vi "Delete Notebook Backup on Quit.vi"(8 "Error In":errorcluster, 11 "Main VI Name":string) -> (0 "Error Out":errorcluster)   [LabVIEW 2019, in "Notebook.lvlib"]
uses:
  Notebook.lvlib
panel:
  # "Check if the Notebook window is open:\nif it is,  don'r do anything.\nif it isn't, delete the backup.\n\nCall this VI when quitting your application."
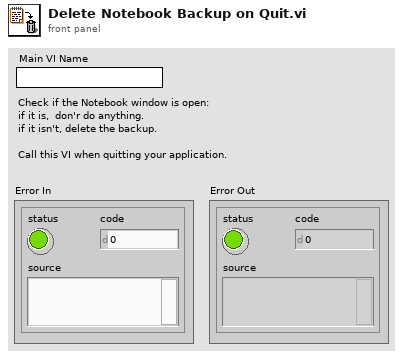
[diagram p1: front panel]
types:
  T1 = enum32{"Invalid", "Standard", "Closed", "Hidden", "Minimized", "Maximized"}
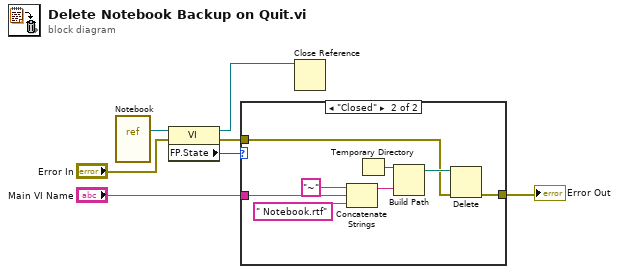
[diagram p0: block diagram]
diagram:
  n1 = vi-ref "Notebook.vi"() -> (w7:refnum<vi>)
  n2 = property class="VI"(reference=w7, error in="Error In") -> (reference out=w4:refnum<vi>, error out=w5:errorcluster, "FP.State"=w6:T1)
  n3 = case shown="\"Closed\"" w6 {
    tunnel: "Main VI Name" -> [_ w12]
    tunnel: w5 -> [w8 w10]
    tunnel: [w8 w9] -> w3
    frame "Invalid", Default {
    }
    frame "Closed" {
      n4 = Concatenate Strings("~" ("string"), w12, " Notebook.rtf" ("format string")) -> (w13:string)
      n5 = Temporary Directory() -> (w16:path)
      n6 = Build Path(base path=w16, name or relative path=w13) -> (appended path=w11:path)
      n7 = Delete(path (use dialog)=w11, error in=w10) -> (error out=w9:errorcluster)  [unwired: 3 in, 2 out]
    }
  }
  "Error Out" <- w3
  n8 = Close Reference(reference=w4) -> ()  [unwired: 1 in, 1 out]
